vi "Configurables.vi"() -> ()   [LabVIEW 2019]
panel:
  out "OldBallHoodOffset(deg)":dbl
  out "AverageBallHoodOffset(deg)":dbl
  out "NewBallHoodOffset(deg)":dbl
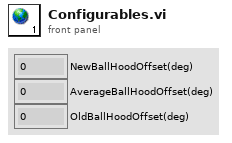
[diagram p1: front panel]
diagram:
